vi "Get Interface.vi"(11 "Plugin in":refnum<class "Dispatcher.lvclass">) -> (2 "Interface":refnum<class "Dispatcher Interface.lvclass">, 3 "Plugin out":refnum<class "Dispatcher.lvclass">)   [LabVIEW 2017, in "DSF Core.lvlib" / "Dispatcher.lvclass"]
uses:
  Dispatcher.lvclass
  Interfaces/Dispatcher/Dispatcher Interface.lvclass
  Dispatcher.lvclass/Dispatcher.ctl
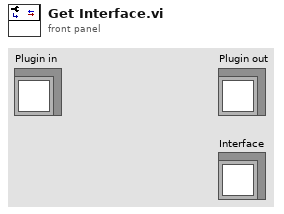
[diagram p1: front panel]
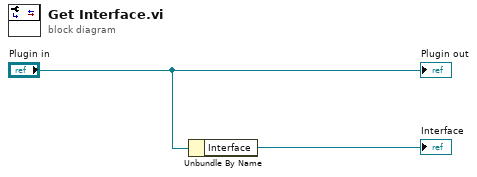
[diagram p0: block diagram]
diagram:
  n1 = Unbundle By Name("Plugin in") -> ("Interface"=→"Interface":refnum<class "Dispatcher Interface.lvclass">)
  "Plugin out" <- "Plugin in"
